vi "Update Default Value Section Visibility.vi"(10 "Previous UI Data in":refnum<class "Settings UI.lvclass">, 11 "New UI Data in":refnum<class "Settings UI.lvclass">) -> (3 "New UI Data out":refnum<class "Settings UI.lvclass">)   [LabVIEW 2024, in "Output Sequencer.lvlib" / "Settings UI.lvclass"]
uses:
  Settings UI.lvclass
  Settings UI.lvclass/Settings UI.ctl
  Types/Tree Index Enum.ctl
  Globals/Global Tree Data.vi
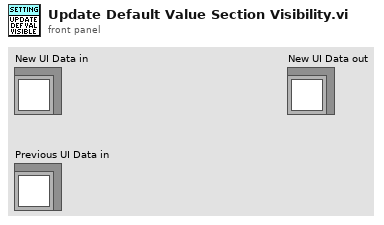
[diagram p1: front panel]
types:
  T1 = typedef "Output Sequencer.lvlib/Settings UI.lvclass/Tree Index Enum.ctl" = enum16{"General Settings", "Num Steps", "Num Analog", "Num Digital", "Show Confirmation", "Interp Priority", "Adv Timing", "Enable Conditions", "Seq Execution", "Reset Test Start", "Only When Test", "Delay After Test", "Start condition", "Re-triggering", "Stop condition", "Stop After Cycles", "Stop Values", "Default Values", "Default Analog", "Default Digital", "Steps", "Step #", "Description", "Precondition", "Duration", "Mode", "Delay Between Vals", "Analog Values", "Digital Values", "Postcondition", "On True", "On False"}
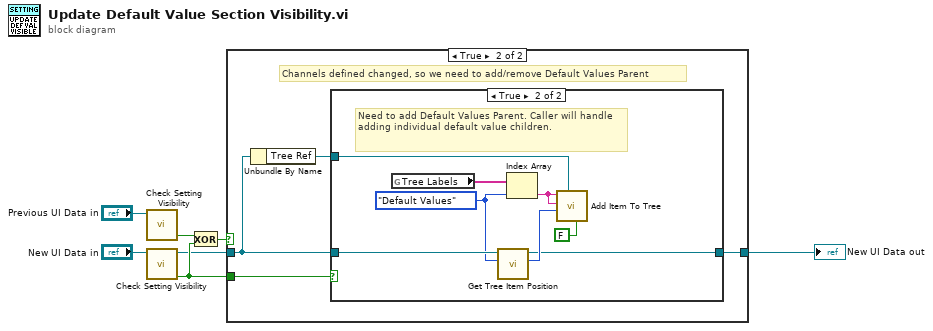
[diagram p0: block diagram]
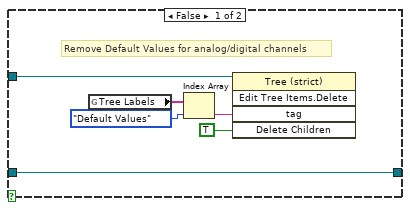
[diagram p3: hidden frame]
diagram:
  n1 = call "Check Setting Visibility.vi"("UI Data in"="Previous UI Data in") -> ("Channels Visible"=w3:bool)  [unwired: 7 in, 3 out]
  n2 = call "Check Setting Visibility.vi"("UI Data in"="New UI Data in") -> ("Channels Visible"=w5:bool, "UI Data out"=w2:refnum<class "Settings UI.lvclass">)  [unwired: 7 in, 2 out]
  n3 = Exclusive Or(1:w5, 2:w3) -> (0:w7:bool)
  n4 = case shown="True" w7 {
    tunnel: w5 -> [_ w12]
    tunnel: w2 -> [w8 w10]
    tunnel: [w8 w11] -> w1
    frame False {
    }
    frame True {
      # "Channels defined changed, so we need to add/remove Default Values Parent"
      n5 = Unbundle By Name(w10) -> ("Tree Ref"=w9:refnum<vi>)
      n6 = case shown="True" w12 {
        tunnel: w9 -> [w15 w26]
        tunnel: w10 -> [w13 w22]
        tunnel: [w13 w19] -> w11
        frame False {
          # "Remove Default Values for analog/digital channels"
          n7 = global read "Global Tree Data.vi" "Tree Labels"() -> (w18:string[])
          n8 = Index Array(array=w18, index=Tree_Index_Enum."Default Values" ("Tree Index Enum")) -> (element=w16:string)
          n9 = invoke class="Tree (strict)" method="Edit Tree Items.Delete"(reference=w15, "tag"=w16, "Delete Children"=TRUE ("Delete Children?")) -> ()  [unwired: 2 in, 5 out]
        }
        frame True {
          w21 = Tree_Index_Enum."Default Values" ("Tree Index Enum")
          # "Need to add Default Values Parent. Caller will handle adding individual default value children."
          n10 = global read "Global Tree Data.vi" "Tree Labels"() -> (w25:string[])
          n11 = call "Get Tree Item Position.vi"("Step item"=w21, "UI Data in"=w22) -> ("Position"=w20:i32, "UI Data out"=w19:refnum<class "Settings UI.lvclass">)  [unwired: 8 in]
          n12 = Index Array(array=w25, index=w21) -> (element=w24:string)
          n13 = call "Add Item To Tree.vi"("Child Only? (true)"=FALSE, "TreeControl in"=w26, "Child Position"=w20, "Left Cell String"=w24, "Child Tag in"=w24) -> ()  [unwired: 6 in, 1 out]
        }
      }
    }
  }
  "New UI Data out" <- w1
